vi "Cannon Get.vi"(1 "Arm?":bool, 2 "Le Fire At Will?":bool) -> ()   [LabVIEW 2013]
uses:
  Cannon Global.vi
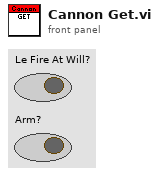
[diagram p1: front panel]
types:
  T1 = typedef "WPI_RelayValue.ctl" = enum16{"Off", "On", "Forward", "Reverse"}
  T2 = cluster{"Angle":dbl, "Clutch MS":bool, "Ball MS":bool, "Motor VBus":dbl, "Clutch ":T1, "LeFireatwill":bool, "Arm":bool, "Armed":bool, "Fire!":bool}
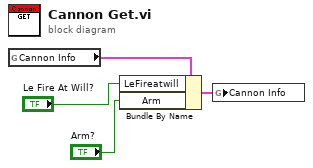
[diagram p0: block diagram]
diagram:
  n1 = global read "Cannon Global.vi" "Cannon Info"() -> (w4:T2)
  n2 = Bundle By Name(cluster=w4, "LeFireatwill"="Le Fire At Will?", "Arm"="Arm?") -> (w3:T2)
  n3 = global write "Cannon Global.vi" "Cannon Info"(w3) -> ()
